vi "Motor Control.vi"(6 "Left":bool, 7 "Right":bool, 9 "Voltage":dbl, 10 "Up":bool, 11 "Down":bool) -> (2 "Motor 1":dbl, 3 "Motor 2":dbl)   [LabVIEW 2015]
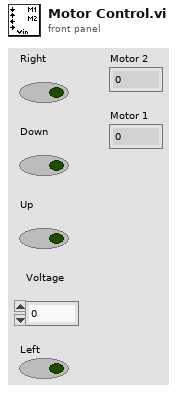
[diagram p1: front panel]
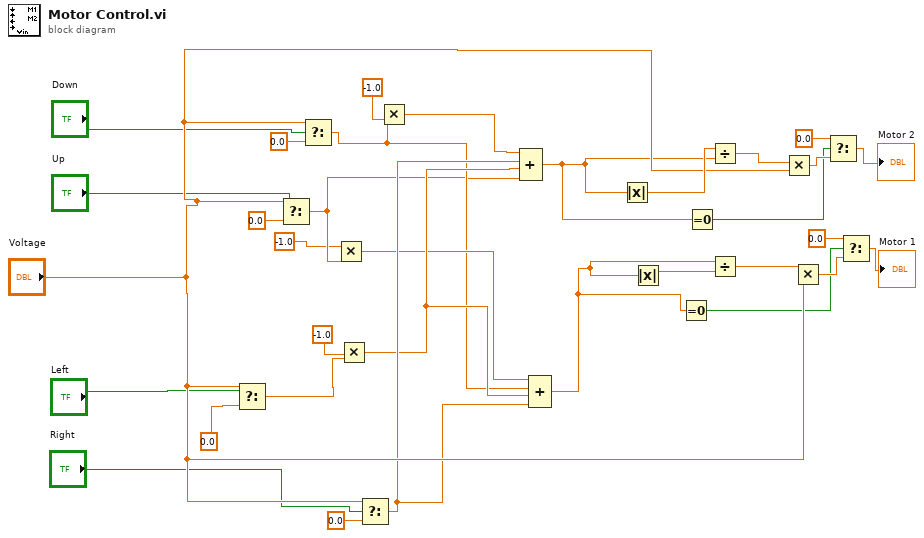
[diagram p0: block diagram]
diagram:
  n1 = Select(t="Voltage", s="Left", f=0.0) -> (s? t:f=w24:dbl)
  n2 = Select(t="Voltage", s="Up", f=0.0) -> (s? t:f=w18:dbl)
  n3 = Select(t="Voltage", s="Down", f=0.0) -> (s? t:f=w25:dbl)
  n4 = Multiply(x=-1.0, y=w18) -> (x*y=w26:dbl)
  n5 = Multiply(x=-1.0, y=w24) -> (x*y=w27:dbl)
  n6 = Select(t="Voltage", s="Right", f=0.0) -> (s? t:f=w28:dbl)
  n7 = Multiply(x=w25, y=-1.0) -> (x*y=w17:dbl)
  n8 = Compound Arithmetic op=ADD(w17, w18, w27, w28) -> (w10:dbl)
  n9 = Compound Arithmetic op=ADD(w26, w25, w27, w28) -> (w3:dbl)
  n10 = Absolute Value(x=w10) -> (abs(x)=w33:dbl)
  n11 = Absolute Value(x=w3) -> (abs(x)=w32:dbl)
  n12 = Equal To 0?(x=w3) -> (x = 0?=w2:bool)
  n13 = Equal To 0?(x=w10) -> (x = 0?=w8:bool)
  n14 = Divide(x=w33, y=w10) -> (x/y=w29:dbl)
  n15 = Divide(x=w3, y=w32) -> (x/y=w30:dbl)
  n16 = Multiply(x=w29, y="Voltage") -> (x*y=w9:dbl)
  n17 = Multiply(x=w30, y="Voltage") -> (x*y=w4:dbl)
  n18 = Select(t=0.0, s=w8, f=w9) -> (s? t:f=→"Motor 2":dbl)
  n19 = Select(t=0.0, s=w2, f=w4) -> (s? t:f=→"Motor 1":dbl)
